vi "Main.vi"() -> ()   [LabVIEW 2024, in "Application.lvlib"]
doc: "This VI is the main application VI in the DQMH project template. This application VI is implemented as a simple state machine, which communicates with two different DQMH modules.\n_____\nBased on DQMH Dev Tools: Project Template 7.1.0.1464."
uses:
  Application.lvlib
  Application Data--cluster.ctl
  State--enum.ctl
  <vilib>/Utility/error.llb/DialogType.ctl
  <vilib>/JKI/JKI Simple Localization/Private/RegisterVIJKI_Simple_Localization.vi
  Cloneable/Cloneable.lvlib
  Singleton/Singleton.lvlib
  <vilib>/JKI/JKI Simple Localization/API/JKI Simple LocalizationJKI_Simple_Localization.lvlib
panel:
  out "Jesus":bool
  in  "DemoLanguage":bool caption="Foco"
  in  "Language ListBox":i32(listbox) caption="Language"
  in  "About DQMH":bool
  out "version":string
  in  "Hide Singleton Module":bool
  in  "Show Singleton Module":bool
  in  "Hide Cloneable Module":bool
  in  "Show Cloneable Module":bool
  in  "Stop Cloneable Module":bool
  in  "Stop Singleton Module":bool
  in  "Start Singleton Module":bool caption="Arrancar Módulo Singleton"
  out "Active Cloneable Modules":string[](array[string]) caption="Clones Activos"
  in  "Start New Instance Cloneable Module":bool
  in  "Select Cloneable Module Instance":i32(ring)=-1 items=["All"=-1]
  in  "Singleton Module: Do Something Else":dbl caption="Do Something Else"
  in  "Singleton Module: Do Something":bool
  out "Singleton Running?":bool caption="Status del Singleton"
  out "Status":string caption="Estado"
  in  "Cloneable Module: Do Something Else":dbl caption="Do Something Else to Selected Module"
  in  "Cloneable Module: Do Something":bool caption="Do Something to Selected Module"
  # "This top-level application allows you to launch and control a singleton module, and multiple instances of a cloneable module."
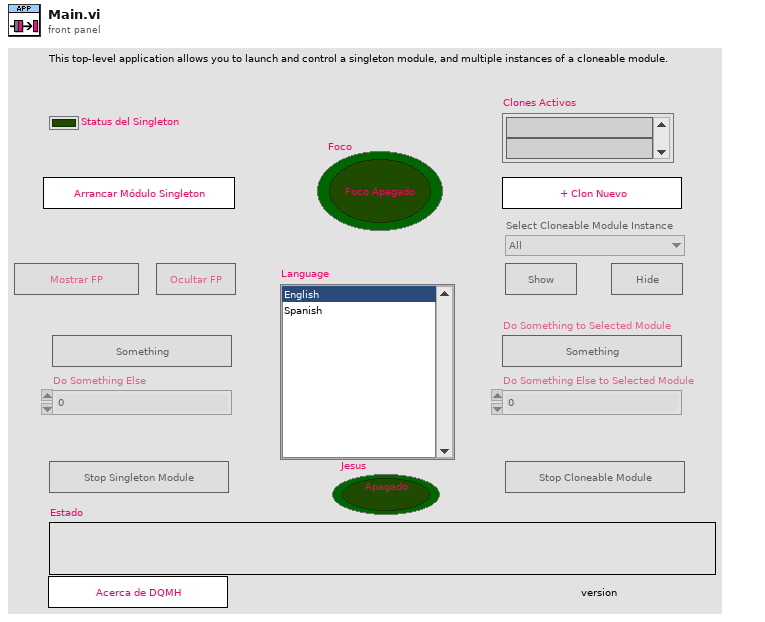
[diagram p1: front panel]
types:
  T1 = typedef "Application.lvlib/State--enum.ctl" = enum16{"Initialize", "Initialize Panel", "UI Interlocks", "Update Status", "Wait for Event", "Exit"}
  T2 = typedef "Application.lvlib/Application Data--cluster.ctl" = cluster{"Status":string, "Singleton Controls":refnum<vi>[], "Cloneable Controls":refnum<vi>[], "Module Ring Value":i32}
  T3 = typedef "Cloneable.lvlib/Broadcast Events--cluster.ctl" = cluster{"Module Did Init":refnum<user-event>, "Status Updated":refnum<user-event>, "Error Reported":refnum<user-event>, "Did Something":refnum<user-event>, "Module Did Stop":refnum<user-event>, "Update Module Execution Status":refnum<user-event>}
  T4 = typedef "Singleton.lvlib/Broadcast Events--cluster.ctl" = cluster{"Module Did Init":refnum<user-event>, "Status Updated":refnum<user-event>, "Error Reported":refnum<user-event>, "Did Something":refnum<user-event>, "Module Did Stop":refnum<user-event>, "Update Module Execution Status":refnum<user-event>}
  T5 = enum8{"Enabled", "Disabled", "Disabled and Grayed Out"}
  T6 = typedef "DialogType.ctl" = u16
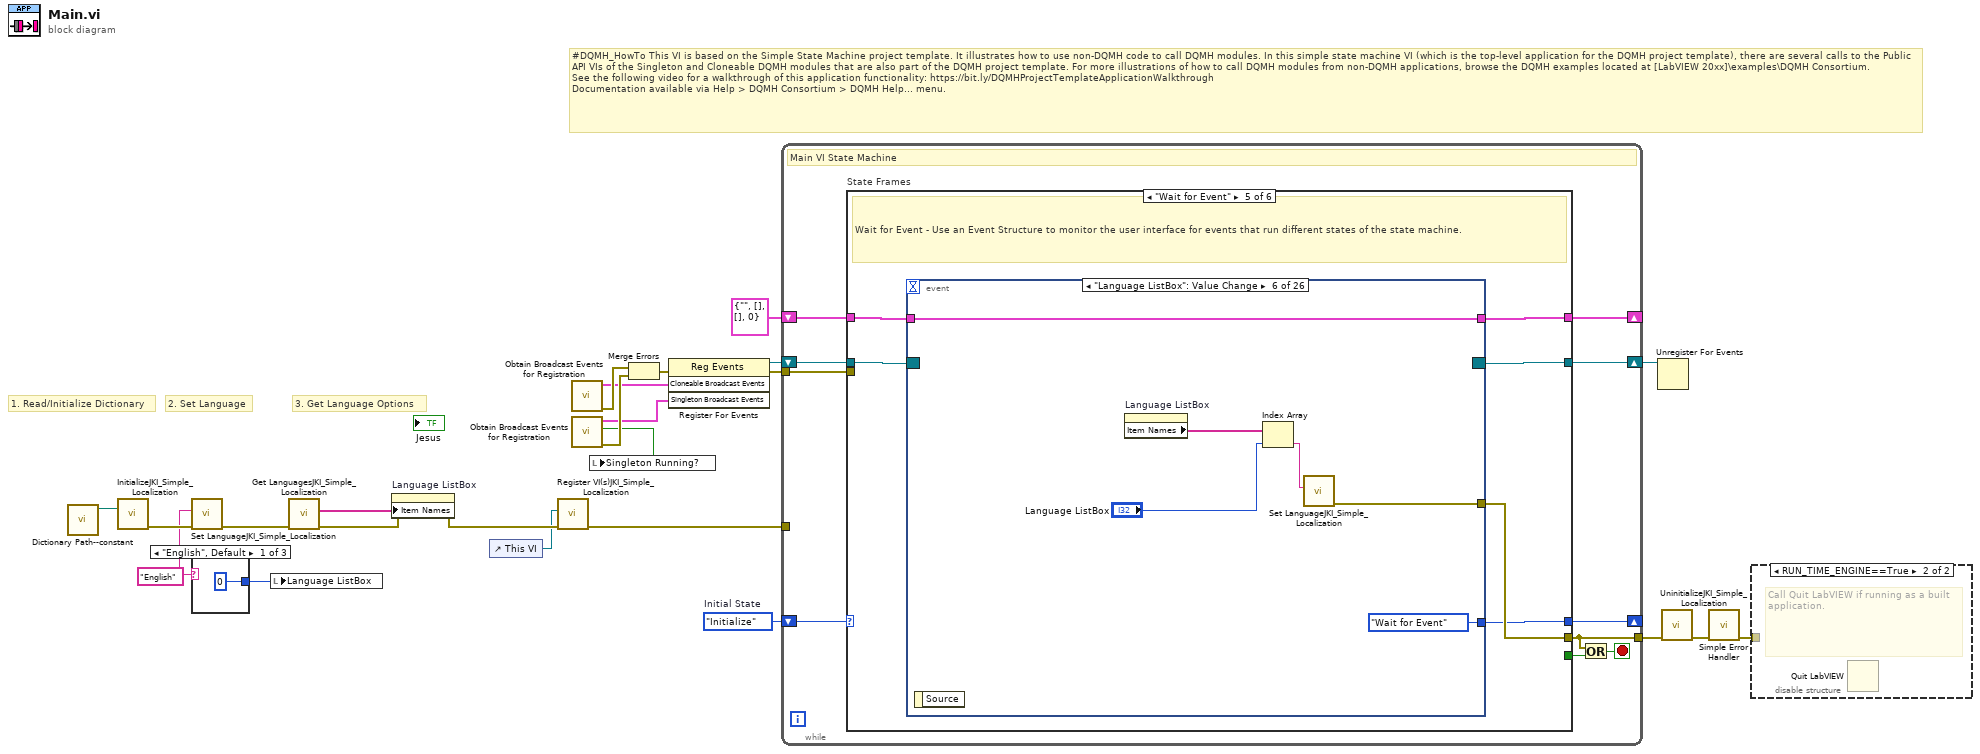
[diagram p0: block diagram]
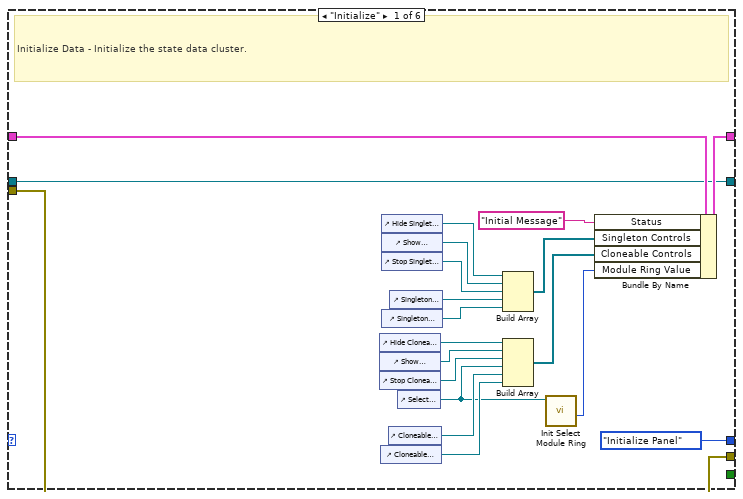
[diagram p2: hidden frame]
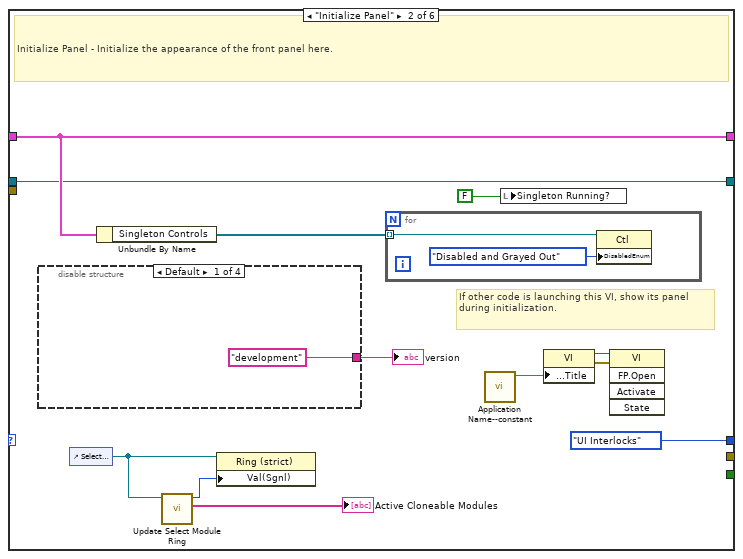
[diagram p3: hidden frame]
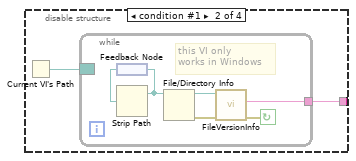
[diagram p4: hidden frame]
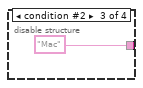
[diagram p5: hidden frame]
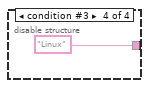
[diagram p6: hidden frame]
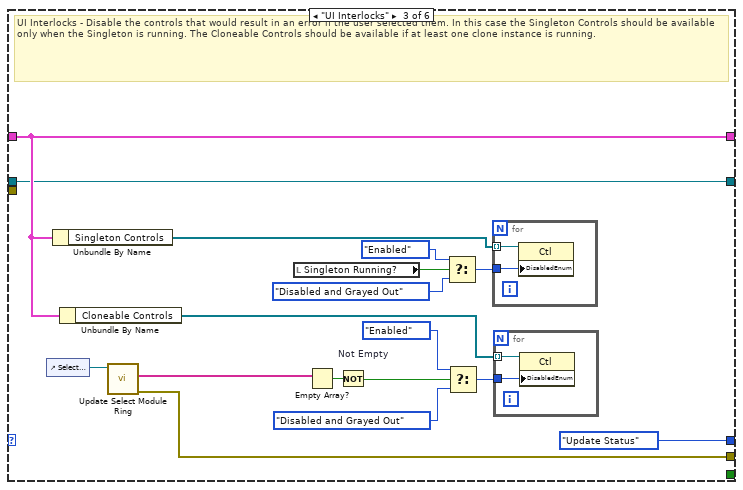
[diagram p7: hidden frame]
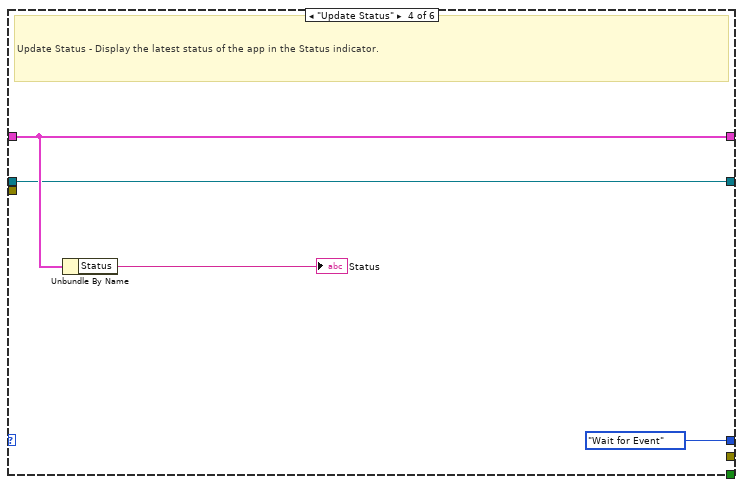
[diagram p8: hidden frame]
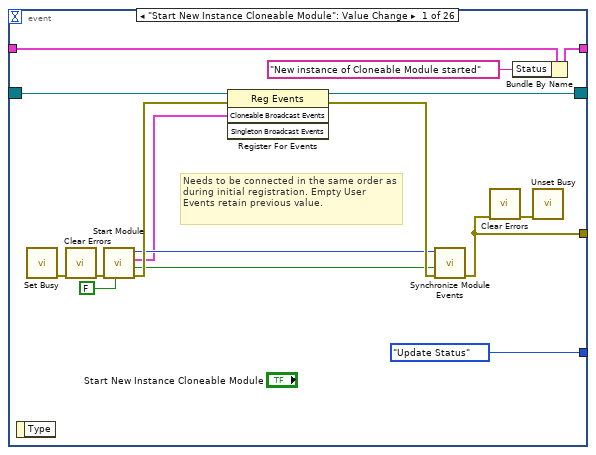
[diagram p9: hidden frame]
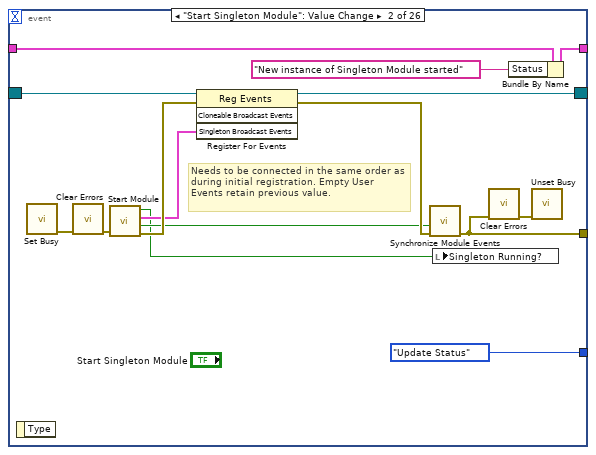
[diagram p10: hidden frame]
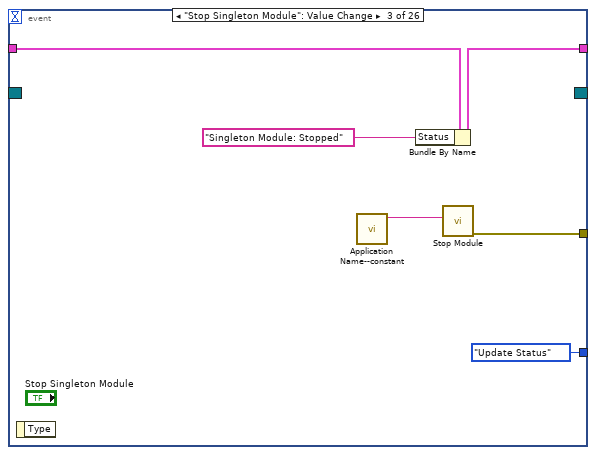
[diagram p11: hidden frame]
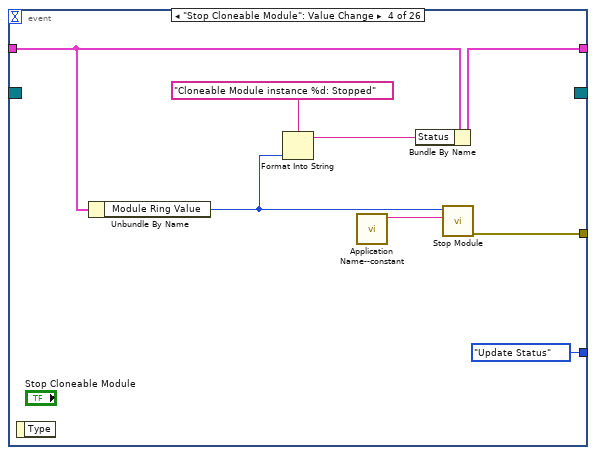
[diagram p12: hidden frame]
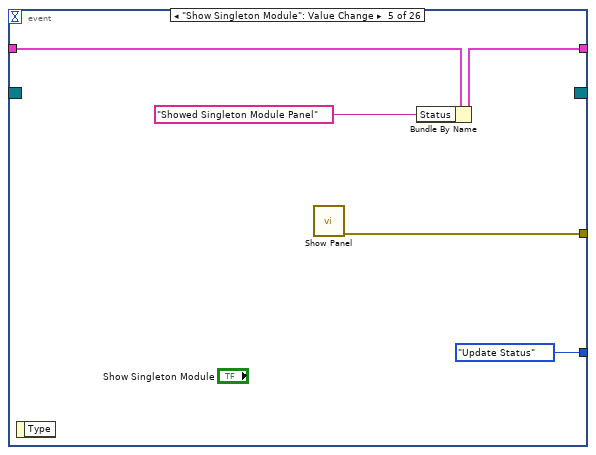
[diagram p13: hidden frame]
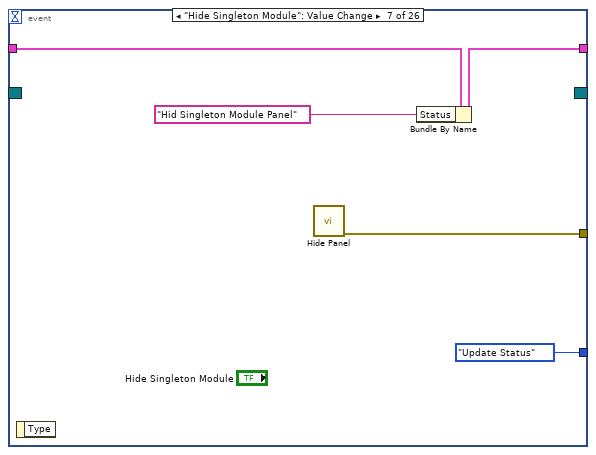
[diagram p14: hidden frame]
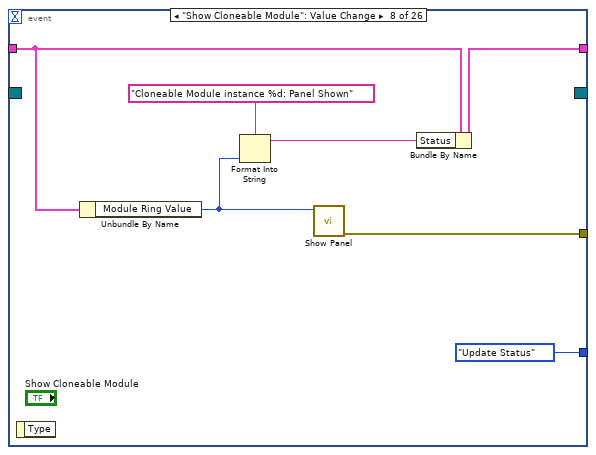
[diagram p15: hidden frame]
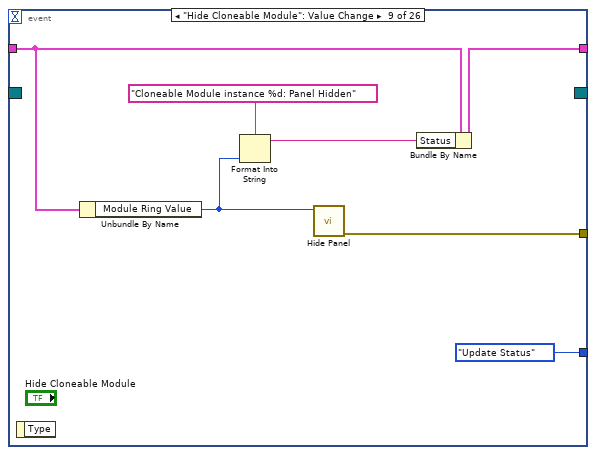
[diagram p16: hidden frame]
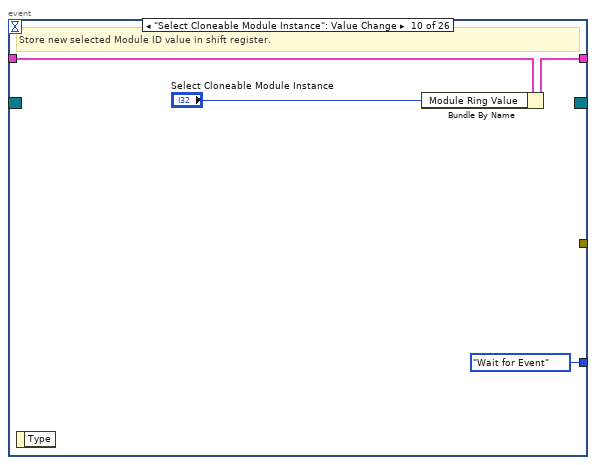
[diagram p17: hidden frame]
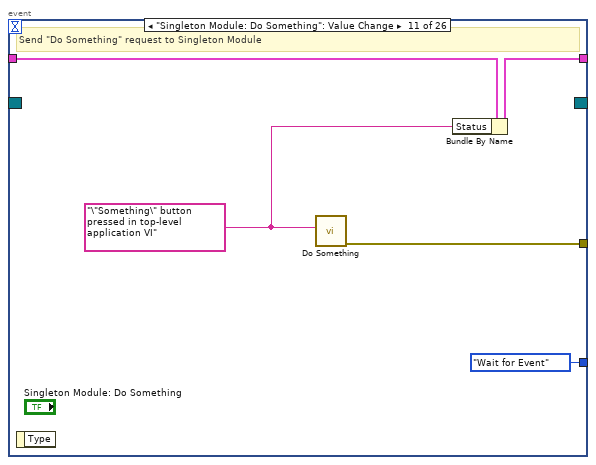
[diagram p18: hidden frame]
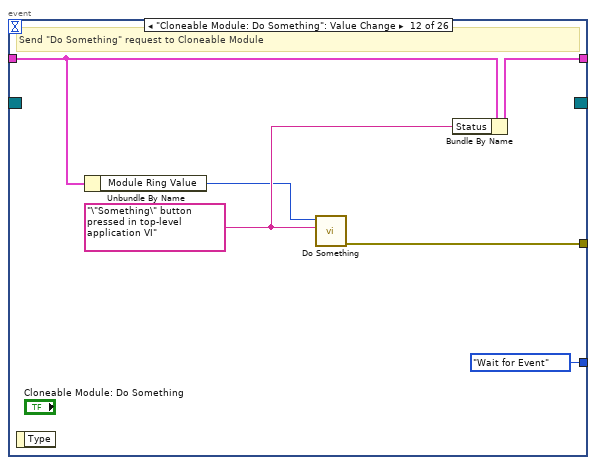
[diagram p19: hidden frame]
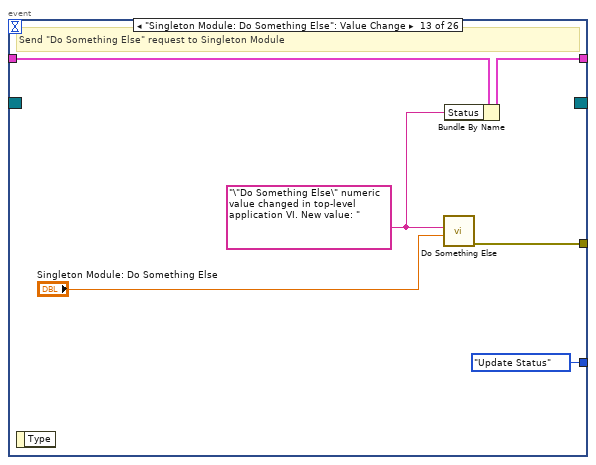
[diagram p20: hidden frame]
diagram:
  w3 = "English" ("Target Language (current lang)")
  w9 = State--enum."Initialize"  # Initial State
  # "3. Get Language Options"
  # "2. Set Language"
  # "1. Read/Initialize Dictionary"
  # "#DQMH_HowTo This VI is based on the Simple State Machine project template. It illustrates how to use non-DQMH code to call DQMH modules. In this simple state machine VI (which is the top-level application for the DQMH project template), there are several calls to the Public API VIs of the Singleton and Cloneable DQMH modules that are also part of the DQMH project template. For more illustrations of how to call DQMH modules from non-DQMH applications, browse the DQMH examples located at [LabVIEW 20xx]\\examples\\DQMH Consortium.\nSee the following video for a walkthrough of this application functionality: https://bit.ly/DQMHProjectTemplateApplicationWalkthrough\nDocumentation available via Help > DQMH Consortium > DQMH Help... menu."
  n1 = call "Dictionary Path--constant.vi"() -> ("appended path"=w2:path)  [unwired: 11 in]
  n2 = call <vilib>:"InitializeJKI_Simple_Localization.vi"("Dictionary File Path"=w2) -> ("error out"=w17:errorcluster)  [unwired: 11 in, 3 out]
  n3 = call <vilib>:"Set LanguageJKI_Simple_Localization.vi"("error in"=w17, "Target Language (current lang)"=w3) -> ("error out"=w16:errorcluster)  [unwired: 8 in, 1 out]
  n4 = case shown="\"English\", Default" w3 {
    tunnel: [0 ("Language ListBox") 1 ("Language ListBox") 3 ("Language ListBox")] -> w4
    frame "English", Default {
    }
    frame "Dutch" {
    }
    frame "Chinese" {
    }
  }
  n5 = local write "Language ListBox"(w4) -> ()
  n6 = call <vilib>:"Get LanguagesJKI_Simple_Localization.vi"("error in"=w16) -> ("error out"=w19:errorcluster, "Languages"=w5:string[])  [unwired: 9 in]
  n7 = property on="Language ListBox" class="LstBox (strict)"(error in=w19, "Item Names"=w5) -> (error out=w18:errorcluster)  [unwired: 1 in, 1 out]
  n8 = control-ref of="This VI"() -> (w1:refnum<vi>)
  n9 = call-poly <vilib>:"Register VI(s)JKI_Simple_Localization.vi"("error in"=w18, "VI Ref"=w1) -> ("error out"=w15:errorcluster)  [unwired: 8 in, 1 out]
  n10 = call "Obtain Broadcast Events for Registration.vi"() -> ("error out"=w21:errorcluster, "Cloneable Broadcast Events"=w11:T3)  [unwired: 9 in, 1 out]
  n11 = call "Obtain Broadcast Events for Registration.vi"() -> ("error out"=w20:errorcluster, "Already running?"=w6:bool, "Singleton Broadcast Events"=w10:T4)  [unwired: 9 in]
  n12 = local write "Singleton Running?"(w6) -> ()
  n13 = Merge Errors(w21, w20) -> (w22:errorcluster)
  n14 = register-events(error in=w22, w11, w10) -> (reference out=w8:refnum<event-registration>, error out=w23:errorcluster)  [unwired: 1 in]
  n15 = while {
    shift-right: [w34] -> _
    shift-left: T2 {"Status"="", "Singleton Controls"=[], "Cloneable Controls"=[], "Module Ring Value"=0} ("Data Cluster") -> [w35]
    tunnel: [w37] -> w14
    shift-right: [w30] -> _
    shift-left: w9 -> [w32]
    shift-right: [w28] -> w7
    shift-left: w8 -> [w29]
    tunnel: w23 -> [w36]
    tunnel: w15 -> [_]
    stop <- w31 stop-if-true
    # "Main VI State Machine"
    n16 = case "State Frames" shown="\"Wait for Event\"" w32 {
      tunnel: [w57 _ w99 _ w113 w300] -> w37
      tunnel: w35 -> [w56 w66 w87 w107 w110 w297]
      tunnel: [w55 w66 w87 w107 w109 w297] -> w34
      tunnel: [_ _ _ _ _ w296] -> w33
      tunnel: [State--enum."Initialize Panel" ("State") State--enum."UI Interlocks" ("State") State--enum."Update Status" ("State") State--enum."Wait for Event" ("State") w108 State--enum."Exit" ("State")] -> w30
      tunnel: w29 -> [w38 w63 w83 w104 w112 w294]
      tunnel: [w38 w63 w83 w104 w111 w294] -> w28
      tunnel: w36 -> [w57 _ _ _ _ _]
      frame "Initialize" {
        # "Initialize Data - Initialize the state data cluster."
        n17 = control-ref of="Hide Cloneable Module"() -> (w47:refnum<vi>)
        n18 = control-ref of="Show Cloneable Module"() -> (w46:refnum<vi>)
        n19 = control-ref of="Stop Cloneable Module"() -> (w45:refnum<vi>)
        n20 = control-ref of="Cloneable Module: Do Something"() -> (w42:refnum<vi>)
        n21 = control-ref of="Hide Singleton Module"() -> (w53:refnum<vi>)
        n22 = control-ref of="Show Singleton Module"() -> (w52:refnum<vi>)
        n23 = control-ref of="Stop Singleton Module"() -> (w51:refnum<vi>)
        n24 = control-ref of="Singleton Module: Do Something"() -> (w49:refnum<vi>)
        n25 = control-ref of="Cloneable Module: Do Something Else"() -> (w43:refnum<vi>)
        n26 = control-ref of="Singleton Module: Do Something Else"() -> (w50:refnum<vi>)
        n27 = control-ref of="Select Cloneable Module Instance"() -> (w40:refnum<vi>)
        n28 = Build Array(w53, w52, w51, w50, w49) -> (w48:refnum<vi>[])
        n29 = Build Array(w47, w46, w45, w40, w43, w42) -> (w44:refnum<vi>[])
        n30 = call "Init Select Module Ring.vi"("Select Module Ring Ref"=w40) -> ("Module Ring Value"=w39:i32)  [unwired: 8 in, 2 out]
        n31 = Bundle By Name(cluster=w56, "Status"="Initial Message" ("Initial Message"), "Singleton Controls"=w48, "Cloneable Controls"=w44, "Module Ring Value"=w39) -> (w55:T2)
      }
      frame "Initialize Panel" {
        # "If other code is launching this VI, show its panel during initialization."
        # "Initialize Panel - Initialize the appearance of the front panel here."
        n32 = disable-structure "Conditional Disable Structure" shown="Default" {
          disable-tunnel: ["development" w71 "Mac" "Linux"] -> w60
          frame condition #0 (active) {
          }
          frame condition #1 {
            n33 = Current VI's Path() -> (path=w72:path)
            n34 = while {
              border: w72 -> [_]
              tunnel: [w73] -> w71
              stop <- w77 continue-if-true
              # "this VI only \nworks in Windows"
              n35 = feedback #1() -> (w76:path)
              n36 = Strip Path(path=w76) -> (stripped path=w75:path)  [unwired: 1 out]
              n37 = feedback-in #1(w75) -> ()
              n38 = File/Directory Info(path=w75) -> (path out=w74:path, error out=w78:errorcluster)  [unwired: 1 in, 5 out]
              n39 = call <vilib>:"FileVersionInfo.vi"("error in (no error)"=w78, "Application Path in"=w74) -> ("error out"=w77:errorcluster, "File Version Info"=w73:string)  [unwired: 6 in, 2 out]
            }
          }
          frame condition #2 {
          }
          frame condition #3 {
          }
        }
        "version" <- w60
        n40 = control-ref of="Select Cloneable Module Instance"() -> (w62:refnum<vi>)
        n41 = Unbundle By Name(w66) -> ("Singleton Controls"=w65:refnum<vi>[])
        n42 = call "Update Select Module Ring.vi"("Select Module Ring Ref"=w62) -> ("Active Modules (Array)"=→"Active Cloneable Modules":string[], "New Module Ring Value"=w61:i32)  [unwired: 8 in, 1 out]
        n43 = property on="Property Node" class="Ring (strict)"(reference=w62, "Val(Sgnl)"=w61) -> ()  [unwired: 1 in, 2 out]
        n44 = for {
          tunnel: w65 -> [w82] mode=indexing
          n45 = property on="Property Node" class="Ctl"(reference=w82, "DisabledEnum"=T5."Disabled and Grayed Out" ("Disabled")) -> ()  [unwired: 1 in, 2 out]
        }
        n46 = call "Application Name--constant.vi"() -> ("Application Name"=w59:string)  [unwired: 11 in]
        n47 = local write "Singleton Running?"(FALSE ("My Singleton Module Init?")) -> ()
        n48 = property on="Property Node" class="VI"("Front Panel.Title"=w59) -> (reference out=w58:refnum<vi>, error out=w69:errorcluster)  [unwired: 2 in]
        n49 = invoke class="VI" method="FP.Open"(reference=w58, error in=w69) -> ()  [unwired: 3 in, 5 out]
      }
      frame "UI Interlocks" {
        # "UI Interlocks - Disable the controls that would result in an error if the user selected them. In this case the Singleton Controls should be available only when the Singleton is running. The Cloneable Controls should be available if at least one clone instance is running."
        n50 = control-ref of="Select Cloneable Module Instance"() -> (w98:refnum<vi>)
        n51 = Unbundle By Name(w87) -> ("Singleton Controls"=w92:refnum<vi>[])
        n52 = Unbundle By Name(w87) -> ("Cloneable Controls"=w86:refnum<vi>[])
        n53 = call "Update Select Module Ring.vi"("Select Module Ring Ref"=w98) -> ("error out"=w99:errorcluster, "Active Modules (Array)"=w97:string[])  [unwired: 8 in, 1 out]
        n54 = local read "Singleton Running?"() -> (w91:bool)
        n55 = Empty Array?(array=w97) -> (empty?=w96:bool)
        n56 = Not "Not Empty"(x=w96) -> (.not. x?=w85:bool)
        n57 = Select(t=T5."Enabled" ("Disabled"), s=w91, f=T5."Disabled and Grayed Out" ("Disabled")) -> (s? t:f=w93:T5)
        n58 = Select(t=T5."Enabled" ("Disabled"), s=w85, f=T5."Disabled and Grayed Out" ("Disabled")) -> (s? t:f=w90:T5)
        n59 = for {
          tunnel: w92 -> [w103] mode=indexing
          tunnel: w93 -> [w102]
          n60 = property on="Property Node" class="Ctl"(reference=w103, "DisabledEnum"=w102) -> ()  [unwired: 1 in, 2 out]
        }
        n61 = for {
          tunnel: w86 -> [w101] mode=indexing
          tunnel: w90 -> [w100]
          n62 = property on="Property Node" class="Ctl"(reference=w101, "DisabledEnum"=w100) -> ()  [unwired: 1 in, 2 out]
        }
      }
      frame "Update Status" {
        # "Update Status - Display the latest status of the app in the Status indicator."
        n63 = Unbundle By Name(w107) -> ("Status"=→"Status":string)
      }
      frame "Wait for Event" {
        # "Wait for Event - Use an Event Structure to monitor the user interface for events that run different states of the state machine."
        n64 = event shown="[5] \"Language ListBox\": Value Change" {
          selector: w112 -> [w121 w137 _ _ _ _ _ _ _ _ _ _ _ _ _ _ _ _ _ _ _ _ _ _ _ _]
          dyn-events: [w120 w136 _ _ _ _ _ _ _ _ _ _ _ _ _ _ _ _ _ _ _ _ _ _ _ _] -> w111
          timeout: _ -> [_ _ _ _ _ _ _ _ _ _ _ _ _ _ _ _ _ _ _ _ _ _ _ _ _ _]
          tunnel: [w129 w144 w150 w158 w163 w169 w174 w181 w188 _ w197 w203 w209 w216 w224 w229 w233 _ _ _ _ w275 _ _ w288 _] -> w113
          tunnel: [w116 w133 w146 w155 w161 w168 w172 w180 w187 w190 w195 w202 w207 w215 w218 w226 w232 w235 w240 w254 w264 w268 w279 w284 w287 w290] -> w109
          tunnel: w110 -> [w117 w134 w147 w154 w162 w168 w173 w178 w185 w191 w196 w199 w208 w213 w218 w226 w232 w236 w241 w255 w265 w271 w280 w284 w287 w290]
          tunnel: [State--enum."Update Status" ("State") State--enum."Update Status" ("State") State--enum."Update Status" ("State") State--enum."Update Status" ("State") State--enum."Update Status" ("State") State--enum."Wait for Event" ("State") State--enum."Update Status" ("State") State--enum."Update Status" ("State") State--enum."Update Status" ("State") State--enum."Wait for Event" ("State") State--enum."Wait for Event" ("State") State--enum."Wait for Event" ("State") State--enum."Update Status" ("State") State--enum."Update Status" ("State") State--enum."UI Interlocks" ("State") State--enum."UI Interlocks" ("State") State--enum."UI Interlocks" ("State") State--enum."Update Status" ("State") State--enum."Update Status" ("State") State--enum."Update Status" ("State") State--enum."Update Status" ("State") State--enum."UI Interlocks" ("State") State--enum."UI Interlocks" ("State") State--enum."Exit" ("State") State--enum."Wait for Event" ("State") State--enum."Wait for Event" ("State")] -> w108
          event "Start New Instance Cloneable Module": Value Change {
            # "Needs to be connected in the same order as during initial registration. Empty User Events retain previous value."
            n65 = event-data() -> ()  [unwired: 1 in, 1 out]
            n66 = call <vilib>:"Set Busy.vi"() -> ("error out"=w125:errorcluster)  [unwired: 10 in, 1 out]
            n67 = call <vilib>:"Clear Errors.vi"("error in (no error)"=w125) -> ("error out"=w126:errorcluster)  [unwired: 5 in, 1 out]
            n68 = call "Start Module.vi"("Show Main VI Diagram on Init (F)"=FALSE, "error in"=w126) -> ("error out"=w128:errorcluster, "Wait for Event Sync?"=w123:bool, "Cloneable Broadcast Events"=w119:T3, "Module ID"=w122:i32)  [unwired: 5 in, 1 out]
            n69 = register-events(reference=w121, error in=w128, w119) -> (reference out=w120:refnum<event-registration>, error out=w127:errorcluster)  [unwired: 1 in]
            n70 = call "Synchronize Module Events.vi"("error in"=w127, "Wait for Event Sync?"=w123, "Module ID in"=w122) -> ("error out"=w129:errorcluster)  [unwired: 7 in, 1 out]
            n71 = call <vilib>:"Clear Errors.vi"("error in (no error)"=w129) -> ("error out"=w124:errorcluster)  [unwired: 5 in, 1 out]
            n72 = Bundle By Name(cluster=w117, "Status"="New instance of Cloneable Module started") -> (w116:T2)
            n73 = call <vilib>:"Unset Busy.vi"("error in (no error)"=w124) -> ()  [unwired: 10 in, 1 out]
          }
          event "Start Singleton Module": Value Change {
            # "Needs to be connected in the same order as during initial registration. Empty User Events retain previous value."
            n74 = event-data() -> ()  [unwired: 1 in, 1 out]
            n75 = call <vilib>:"Set Busy.vi"() -> ("error out"=w140:errorcluster)  [unwired: 10 in, 1 out]
            n76 = call <vilib>:"Clear Errors.vi"("error in (no error)"=w140) -> ("error out"=w141:errorcluster)  [unwired: 5 in, 1 out]
            n77 = call "Start Module.vi"("error in"=w141) -> ("error out"=w143:errorcluster, "Wait for Event Sync?"=w138:bool, "Singleton Broadcast Events"=w131:T4, "Module Was Already Running?"=w130:bool)  [unwired: 6 in, 1 out]
            n78 = register-events(reference=w137, error in=w143, w131) -> (reference out=w136:refnum<event-registration>, error out=w142:errorcluster)  [unwired: 1 in]
            n79 = call "Synchronize Module Events.vi"("error in"=w142, "Wait for Event Sync?"=w138) -> ("error out"=w144:errorcluster)  [unwired: 9 in]
            n80 = local write "Singleton Running?"(w130) -> ()
            n81 = call <vilib>:"Clear Errors.vi"("error in (no error)"=w144) -> ("error out"=w139:errorcluster)  [unwired: 5 in, 1 out]
            n82 = Bundle By Name(cluster=w134, "Status"="New instance of Singleton Module started") -> (w133:T2)
            n83 = call <vilib>:"Unset Busy.vi"("error in (no error)"=w139) -> ()  [unwired: 10 in, 1 out]
          }
          event "Stop Singleton Module": Value Change {
            n84 = event-data() -> ()  [unwired: 1 in, 1 out]
            n85 = call "Application Name--constant.vi"() -> ("Application Name"=w148:string)  [unwired: 11 in]
            n86 = Bundle By Name(cluster=w147, "Status"="Singleton Module: Stopped" ("Message")) -> (w146:T2)
            n87 = call "Stop Module.vi"("Origin"=w148) -> ("error out"=w150:errorcluster)  [unwired: 10 in]
          }
          event "Stop Cloneable Module": Value Change {
            n88 = event-data() -> ()  [unwired: 1 in, 1 out]
            n89 = Unbundle By Name(w154) -> ("Module Ring Value"=w151:i32)
            n90 = Format Into String(format string="Cloneable Module instance %d: Stopped" ("Message"), w151) -> (resulting string=w152:string)  [unwired: 2 in, 1 out]
            n91 = call "Application Name--constant.vi"() -> ("Application Name"=w156:string)  [unwired: 11 in]
            n92 = Bundle By Name(cluster=w154, "Status"=w152) -> (w155:T2)
            n93 = call "Stop Module.vi"("Origin"=w156, "Module ID"=w151) -> ("error out"=w158:errorcluster)  [unwired: 9 in]
          }
          event "Show Singleton Module": Value Change {
            n94 = event-data() -> ()  [unwired: 1 in, 1 out]
            n95 = call "Show Panel.vi"() -> ("error out"=w163:errorcluster)  [unwired: 11 in]
            n96 = Bundle By Name(cluster=w162, "Status"="Showed Singleton Module Panel" ("Message")) -> (w161:T2)
          }
          event "Language ListBox": Value Change {
            n97 = event-data() -> ()  [unwired: 1 in, 1 out]
            n98 = property on="Language ListBox" class="LstBox (strict)"() -> ("Item Names"=w167:string[])  [unwired: 2 in, 2 out]
            n99 = Index Array(array=w167, index="Language ListBox") -> (element=w165:string)
            n100 = call <vilib>:"Set LanguageJKI_Simple_Localization.vi"("Target Language (current lang)"=w165) -> ("error out"=w169:errorcluster)  [unwired: 9 in, 1 out]
          }
          event "Hide Singleton Module": Value Change {
            n101 = event-data() -> ()  [unwired: 1 in, 1 out]
            n102 = call "Hide Panel.vi"() -> ("error out"=w174:errorcluster)  [unwired: 11 in]
            n103 = Bundle By Name(cluster=w173, "Status"="Hid Singleton Module Panel" ("Message")) -> (w172:T2)
          }
          event "Show Cloneable Module": Value Change {
            n104 = event-data() -> ()  [unwired: 1 in, 1 out]
            n105 = Unbundle By Name(w178) -> ("Module Ring Value"=w176:i32)
            n106 = Format Into String(format string="Cloneable Module instance %d: Panel Shown" ("Message"), w176) -> (resulting string=w175:string)  [unwired: 2 in, 1 out]
            n107 = call "Show Panel.vi"("Module ID"=w176) -> ("error out"=w181:errorcluster)  [unwired: 10 in]
            n108 = Bundle By Name(cluster=w178, "Status"=w175) -> (w180:T2)
          }
          event "Hide Cloneable Module": Value Change {
            n109 = event-data() -> ()  [unwired: 1 in, 1 out]
            n110 = Unbundle By Name(w185) -> ("Module Ring Value"=w183:i32)
            n111 = Format Into String(format string="Cloneable Module instance %d: Panel Hidden" ("Message"), w183) -> (resulting string=w182:string)  [unwired: 2 in, 1 out]
            n112 = call "Hide Panel.vi"("Module ID"=w183) -> ("error out"=w188:errorcluster)  [unwired: 10 in]
            n113 = Bundle By Name(cluster=w185, "Status"=w182) -> (w187:T2)
          }
          event "Select Cloneable Module Instance": Value Change {
            # "Store new selected Module ID value in shift register."
            n114 = event-data() -> ()  [unwired: 1 in, 1 out]
            n115 = Bundle By Name(cluster=w191, "Module Ring Value"="Select Cloneable Module Instance") -> (w190:T2)
          }
          event "Singleton Module: Do Something": Value Change {
            w194 = "\"Something\" button pressed in top-level application VI" ("\"Do Something Else\" button pressed")
            # "Send \"Do Something\" request to Singleton Module"
            n116 = event-data() -> ()  [unwired: 1 in, 1 out]
            n117 = call "Do Something.vi"("Do Something Message"=w194) -> ("error out"=w197:errorcluster)  [unwired: 10 in]
            n118 = Bundle By Name(cluster=w196, "Status"=w194) -> (w195:T2)
          }
          event "Cloneable Module: Do Something": Value Change {
            w201 = "\"Something\" button pressed in top-level application VI" ("\"Do Something Else\" button pressed")
            # "Send \"Do Something\" request to Cloneable Module"
            n119 = event-data() -> ()  [unwired: 1 in, 1 out]
            n120 = Unbundle By Name(w199) -> ("Module Ring Value"=w198:i32)
            n121 = call "Do Something.vi"("Do Something Message"=w201, "Module ID"=w198) -> ("error out"=w203:errorcluster)  [unwired: 9 in]
            n122 = Bundle By Name(cluster=w199, "Status"=w201) -> (w202:T2)
          }
          event "Singleton Module: Do Something Else": Value Change {
            w204 = "\"Do Something Else\" numeric value changed in top-level application VI. New value: " ("\"Do Something Else\" button pressed")
            # "Send \"Do Something Else\" request to Singleton Module"
            n123 = event-data() -> ()  [unwired: 1 in, 1 out]
            n124 = call "Do Something Else.vi"("X"="Singleton Module: Do Something Else", "Do Something Else Message"=w204) -> ("error out"=w209:errorcluster)  [unwired: 9 in]
            n125 = Bundle By Name(cluster=w208, "Status"=w204) -> (w207:T2)
          }
          event "Cloneable Module: Do Something Else": Value Change {
            w210 = "\"Do Something Else\" numeric value changed in top-level application VI. New value: " ("\"Do Something Else\" button pressed")
            # "Send \"Do Something Else\" request to Cloneable Module"
            n126 = event-data() -> ()  [unwired: 1 in, 1 out]
            n127 = Unbundle By Name(w213) -> ("Module Ring Value"=w212:i32)
            n128 = call "Do Something Else.vi"("X"="Cloneable Module: Do Something Else", "Do Something else Message"=w210, "Module ID"=w212) -> ("error out"=w216:errorcluster)  [unwired: 8 in]
            n129 = Bundle By Name(cluster=w213, "Status"=w210) -> (w215:T2)
          }
          event User Event {
            # "A new instance of Cloneable Module has broadcast that is has been initialized"
            n130 = event-data() -> ("Info"=w222:string, "Module ID"=w217:i32)  [unwired: 1 in]
            n131 = local write "Status"(w222) -> ()
            n132 = control-ref of="Select Cloneable Module Instance"() -> (w221:refnum<vi>)
            n133 = call "Update Select Module Ring.vi"("Select Module Ring Ref"=w221) -> ("error out"=w223:errorcluster, "Active Modules (Array)"=w220:string[])  [unwired: 8 in, 1 out]
            n134 = local write "Active Cloneable Modules"(w220) -> ()
            n135 = call "Show Panel.vi"("error in"=w223, "Module ID"=w217) -> ("error out"=w224:errorcluster)  [unwired: 9 in]
          }
          event User Event {
            # "Singleton Module has broadcast that it has been initialized"
            n136 = event-data() -> ("Init?"=→"Singleton Running?":bool, "Info"=w228:string)  [unwired: 1 in]
            n137 = local write "Status"(w228) -> ()
            n138 = call "Show Panel.vi"() -> ("error out"=w229:errorcluster)  [unwired: 11 in]
          }
          event User Event {
            # "Singleton Module has broadcast its execution status"
            n139 = event-data() -> ("Running?"=w230:bool)  [unwired: 1 in]
            n140 = local write "Singleton Running?"(w230) -> ()
            n141 = case shown="True" w230 {
              tunnel: [_ w234] -> w233
              frame False {
              }
              frame True {
                n142 = call "Show Panel.vi"() -> ("error out"=w234:errorcluster)  [unwired: 11 in]
              }
            }
          }
          event User Event {
            # "An instance of Cloneable Module has broadcast its status"
            n143 = event-data() -> ("Status"=w238:string)  [unwired: 1 in]
            n144 = Bundle By Name(cluster=w236, "Status"=w238) -> (w235:T2)
          }
          event User Event {
            # "Singleton Module has broadcast its status"
            n145 = event-data() -> ("Status"=w242:string)  [unwired: 1 in]
            n146 = Bundle By Name(cluster=w241, "Status"=w242) -> (w240:T2)
          }
          event User Event {
            w246 = T6 0 items=["no dialog", "OK message", "continue or stop message", "OK message + warnings", "continue/stop + warnings"] ("type of dialog (OK msg:1)")
            # "Cloneable Module had an error"
            n147 = event-data() -> ("Module Name"=w244:string, "Additional Information"=w245:string, "Error"=w256:errorcluster)  [unwired: 1 in]
            n148 = call <vilib>:"Space Constant.vi"() -> ("String"=w250:string)
            n149 = call <vilib>:"Simple Error Handler.vi"("type of dialog (OK msg:1)"=w246, "error in (no error)"=w256) -> ("message"=w247:string)  [unwired: 3 in, 4 out]
            n150 = call <vilib>:"Search and Replace Pattern.vi"("string"=w247, "regular expression (\"\")"="[\\r\\n]" ("regular expression (\"\")"), "replace string (\"\")"=w250, "replace all? (F)"=TRUE ("replace all CR/LF with spaces")) -> ("result string"=w248:string)  [unwired: 1 in, 1 out]
            n151 = Format Into String(format string="%s: %s Additional Information: %s", w244, w248, w245) -> (resulting string=w243:string)  [unwired: 2 in, 1 out]
            n152 = Bundle By Name(cluster=w255, "Status"=w243) -> (w254:T2)
          }
          event User Event {
            # "Singleton Module had an error"
            n153 = event-data() -> ("Module Name"=w258:string, "Additional Information"=w262:string, "Error"=w266:errorcluster)  [unwired: 1 in]
            n154 = Unbundle By Name(w266) -> ("code"=w257:i32, "source"=w261:string)
            n155 = Format Into String(format string="Error code %d Module: %s  Additional Information: %s\nSource: %s", w257, w258, w262, w261) -> (resulting string=w259:string)  [unwired: 2 in, 1 out]
            n156 = Bundle By Name(cluster=w265, "Status"=w259) -> (w264:T2)
          }
          event User Event {
            n157 = event-data() -> ("Origin"=w270:string)  [unwired: 1 in]
            n158 = Bundle By Name(cluster=w271, "Status"=w270) -> (w269:T2)
            n159 = control-ref of="Select Cloneable Module Instance"() -> (w274:refnum<vi>)
            n160 = call "Update Select Module Ring.vi"("Select Module Ring Ref"=w274) -> ("error out"=w275:errorcluster, "Active Modules (Array)"=w273:string[], "New Module Ring Value"=w267:i32)  [unwired: 8 in]
            n161 = Bundle By Name(cluster=w269, "Module Ring Value"=w267) -> (w268:T2)
            n162 = local write "Active Cloneable Modules"(w273) -> ()
          }
          event User Event {
            n163 = event-data() -> ("Origin"=w277:string)  [unwired: 1 in]
            n164 = local write "Singleton Running?"(FALSE ("My Singleton Module Init?")) -> ()
            n165 = Concatenate Strings(w277, " Did Stop.") -> (w276:string)
            n166 = Bundle By Name(cluster=w280, "Status"=w276) -> (w279:T2)
          }
          event Panel Close? {
            # "Go to the 'Exit' state if the user tries to close the panel."
            n167 = event-data() -> ()  [unwired: 1 in, 1 out]
            n168 = event-data ("Event Filter Node")("Discard?"=TRUE) -> ()  [unwired: 1 in, 1 out]
          }
          event "About DQMH": Value Change {
            # "Display DQMH About Box"
            n169 = event-data() -> ()  [unwired: 1 in, 1 out]
            n170 = call <vilib>:"DQMH_About Box.vi"() -> ("error out"=w288:errorcluster)  [unwired: 11 in]
          }
          event "DemoLanguage": Value Change {
            n171 = event-data() -> ()  [unwired: 1 in, 1 out]
          }
        }
      }
      frame "Exit" {
        w291 = TRUE  # Wait for Module to stop?
        w296 = TRUE  # Stop the VI
        # "Stop all modules launched"
        # "Exit - Exit the application."
        n172 = call "Application Name--constant.vi"() -> ("Application Name"=w292:string)  [unwired: 11 in]
        n173 = call "Stop Module.vi"("Wait for Module to stop? (F)"=w291, "Origin"=w292, "Module ID"=-1) -> ("error out"=w298:errorcluster)  [unwired: 8 in]
        n174 = call "Stop Module.vi"("Wait for Module to Stop? (F)"=w291, "Origin"=w292) -> ("error out"=w299:errorcluster)  [unwired: 9 in]
        n175 = Merge Errors(w298, w299) -> (w300:errorcluster)
      }
    }
    n176 = Or(x=w37, y=w33) -> (x .or. y?=w31:bool)
  }
  n177 = Unregister For Events(event registration refnum=w7) -> ()  [unwired: 1 in, 1 out]
  n178 = call <vilib>:"UninitializeJKI_Simple_Localization.vi"("error in"=w14) -> ("error out"=w13:errorcluster)  [unwired: 10 in]
  n179 = call <vilib>:"Simple Error Handler.vi"("error in (no error)"=w13) -> ("error out"=w24:errorcluster)  [unwired: 4 in, 4 out]
  n180 = disable-structure "Conditional Disable Structure" shown="RUN_TIME_ENGINE==True" {
    disable-tunnel: w24 -> [_ _]
    frame condition #0 (active) {
    }
    frame condition #1 {
      # "Call Quit LabVIEW if running as a built application."
      n181 = Quit LabVIEW() -> ()  [unwired: 1 in]
    }
  }
